vi "Vertical Insert.vi"(4 "Side":T1=enum."right", 8 "error in":errorcluster, 9 "Speed":dbl=10.0, 10 "depth":dbl) -> (0 "error out":errorcluster)   [LabVIEW 2013]
uses:
  ROS/Code/SubVIs/BaxterSide.ctl
  ROS/Code/Console/Servers/ServerSubs/(nist) Arm Globals.vi
  Prim/Fwd Kenimatics - array.vi
  <vilib>/Analysis/Matrix/Numeric/Multiply/Multiply - RM,RM.vi
  Move Matrix.vi
  <vilib>/Analysis/Matrix/NI_Matrix.lvlib
panel:
  in  "MaxAngle":dbl=40.0
  in  "deg/mm":dbl=10.0
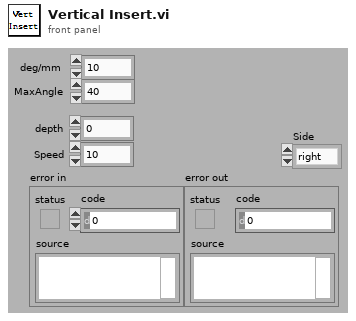
[diagram p1: front panel]
types:
  T1 = typedef "BaxterSide.ctl" = enum16{"left", "right"}
  T2 = cluster{"X":dbl, "Y":dbl, "Z":dbl, "Roll":dbl, "Pitch":dbl, "Yaw":dbl}
  T3 = typedef "NI_Matrix.lvlib/RealMatrix.ctl" = dbl[][]
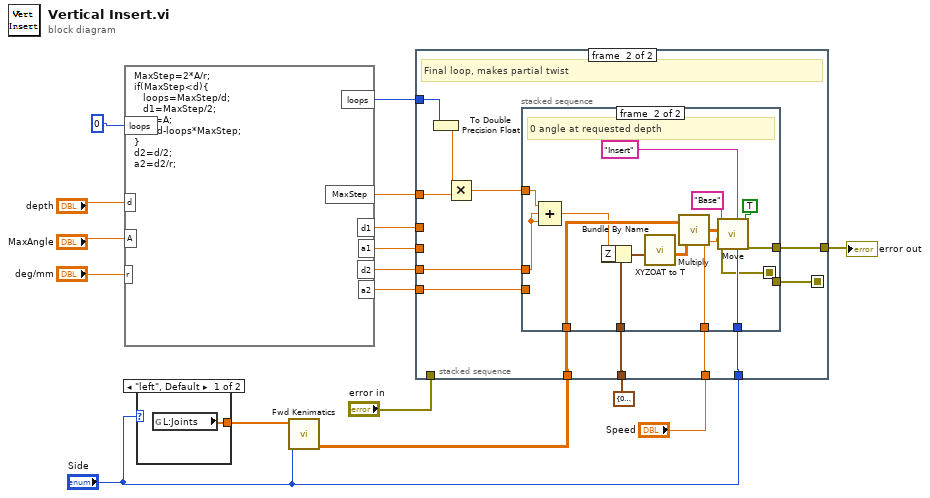
[diagram p0: block diagram]
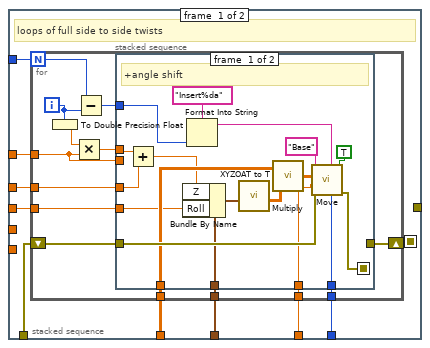
[diagram p2: hidden frame]
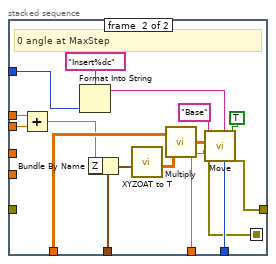
[diagram p3: hidden frame]
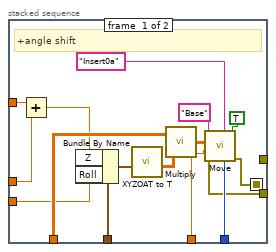
[diagram p4: hidden frame]
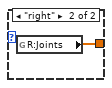
[diagram p5: hidden frame]
diagram:
  n1 = formula code="MaxStep=2*A/r;\nif(MaxStep<d){\n   loops=MaxStep/d;\n   d1=MaxStep/2;\n   a1=A;\n   d=d-loops*MaxStep;\n}\nd2=d/2;\na2=d2/r;"("d"="depth", "A"="MaxAngle", "r"="deg/mm", "loops"=0) -> ("MaxStep"=w5:dbl, "loops"=w13:i32, "d1"=w12:dbl, "a1"=w11:dbl, "d2"=w2:dbl, "a2"=w3:dbl)
  n2 = case shown="\"left\", Default" "Side" {
    tunnel: [w18 w19] -> w17
    frame "left", Default {
      n3 = global read "(nist) Arm Globals.vi" "L:Joints"() -> (w18:dbl[])
    }
    frame "right" {
      n4 = global read "(nist) Arm Globals.vi" "R:Joints"() -> (w19:dbl[])
    }
  }
  n5 = call-poly "Fwd Kenimatics.vi"("Side"="Side", "Joints"=w17) -> ("Matrix"=w9:T3)  [unwired: 8 in, 1 out]
  n6 = stacked-sequence {
    seq-local: [w20 _] -> [_ w83]
    tunnel: w13 -> [w29 w90]
    tunnel: w12 -> [w28 _]
    tunnel: w11 -> [w27 _]
    tunnel: "error in" -> [w26 _]
    tunnel: w9 -> [w25 w84]
    tunnel: T2 {"X"=0.0, "Y"=0.0, "Z"=0.0, "Roll"=0.0, "Pitch"=0.0, "Yaw"=0.0} ("XYZOAT") -> [w24 w81]
    tunnel: "Speed" -> [w23 w82]
    tunnel: "Side" -> [w22 w80]
    tunnel: w5 -> [w21 w89]
    tunnel: w3 -> [_ w87]
    tunnel: w2 -> [_ w86]
    tunnel: [_ w79] -> w1
    frame #0 {
      # "loops of full side to side twists"
      n7 = for {
        N: w29 -> [w32]
        tunnel: w28 -> [w34]
        tunnel: w27 -> [w39]
        shift-right: [w42] -> w20
        shift-left: w26 -> [w43]
        tunnel: w25 -> [w41]
        tunnel: w24 -> [w40]
        tunnel: w23 -> [w38]
        tunnel: w22 -> [w37]
        tunnel: w21 -> [w33]
        i -> [w31]
        n8 = To Double Precision Float(number=w31) -> (double precision float=w36:dbl)
        n9 = Multiply(x=w36, y=w33) -> (x*y=w35:dbl)
        n10 = Subtract(x=w32, y=w31) -> (x-y=w30:i32)
        n11 = stacked-sequence {
          seq-local: [w44 _] -> [_ w66]
          tunnel: w43 -> [w61 _]
          tunnel: w30 -> [w58 w76]
          tunnel: [_ w65] -> w42
          tunnel: w41 -> [w56 w74]
          tunnel: w40 -> [w52 w70]
          tunnel: w39 -> [w48 _]
          tunnel: w38 -> [w50 w68]
          tunnel: w37 -> [w49 w67]
          tunnel: w35 -> [w47 w64]
          tunnel: w34 -> [w46 _]
          tunnel: w33 -> [_ w63]
          frame #0 {
            # "+angle shift"
            n12 = Add(x=w47, y=w46) -> (x+y=w45:dbl)
            n13 = Bundle By Name(cluster=w52, "Z"=w45, "Roll"=w48) -> (w53:T2)
            n14 = Format Into String(format string="Insert%da", w58) -> (resulting string=w57:string)  [unwired: 2 in, 1 out]
            n15 = call "XYZOAT to T.vi"("XYZOAT"=w53) -> ("T"=w54:T3)  [unwired: 10 in]
            n16 = call-poly <vilib>:"Multiply.vi"("Real Matrix B"=w54, "Real Matrix A"=w56) -> ("A * B"=w55:T3)
            n17 = call-poly "Move.vi"("Make Vertical"=TRUE, "Side"=w49, "Label"=w57, "error in"=w61, "Speed (mm/s)"=w50, "Offset"=w55, "Location"="Base") -> ("error out"=w44:errorcluster)  [unwired: 4 in]
          }
          frame #1 {
            # "0 angle at MaxStep"
            n18 = Add(x=w64, y=w63) -> (x+y=w62:dbl)
            n19 = Format Into String(format string="Insert%dc", w76) -> (resulting string=w75:string)  [unwired: 2 in, 1 out]
            n20 = Bundle By Name(cluster=w70, "Z"=w62) -> (w71:T2)
            n21 = call "XYZOAT to T.vi"("XYZOAT"=w71) -> ("T"=w72:T3)  [unwired: 10 in]
            n22 = call-poly <vilib>:"Multiply.vi"("Real Matrix B"=w72, "Real Matrix A"=w74) -> ("A * B"=w73:T3)
            n23 = call-poly "Move.vi"("Make Vertical"=TRUE, "Side"=w67, "Label"=w75, "error in"=w66, "Speed (mm/s)"=w68, "Offset"=w73, "Location"="Base") -> ("error out"=w65:errorcluster)  [unwired: 4 in]
          }
        }
      }
    }
    frame #1 {
      # "Final loop, makes partial twist"
      n24 = To Double Precision Float(number=w90) -> (double precision float=w88:dbl)
      n25 = Multiply(x=w88, y=w89) -> (x*y=w85:dbl)
      n26 = stacked-sequence {
        seq-local: [w93 _] -> [_ w112]
        tunnel: [_ w111] -> w79
        tunnel: w84 -> [w105 w120]
        tunnel: w81 -> [w101 w116]
        tunnel: w87 -> [w97 _]
        tunnel: w82 -> [w99 w114]
        tunnel: w80 -> [w98 w113]
        tunnel: w85 -> [w96 w110]
        tunnel: w86 -> [w95 w108]
        tunnel: w83 -> [w91 _]
        frame #0 {
          # "+angle shift"
          n27 = Add(x=w96, y=w95) -> (x+y=w94:dbl)
          n28 = Bundle By Name(cluster=w101, "Z"=w94, "Roll"=w97) -> (w102:T2)
          n29 = call "XYZOAT to T.vi"("XYZOAT"=w102) -> ("T"=w103:T3)  [unwired: 10 in]
          n30 = call-poly <vilib>:"Multiply.vi"("Real Matrix B"=w103, "Real Matrix A"=w105) -> ("A * B"=w104:T3)
          n31 = call-poly "Move.vi"("Make Vertical"=TRUE, "Side"=w98, "Label"="Insert0a" ("format string"), "error in"=w91, "Speed (mm/s)"=w99, "Offset"=w104, "Location"="Base") -> ("error out"=w93:errorcluster)  [unwired: 4 in]
        }
        frame #1 {
          # "0 angle at requested depth"
          n32 = Compound Arithmetic op=ADD(w110, w108, w108) -> (w109:dbl)
          n33 = Bundle By Name(cluster=w116, "Z"=w109) -> (w117:T2)
          n34 = call "XYZOAT to T.vi"("XYZOAT"=w117) -> ("T"=w118:T3)  [unwired: 10 in]
          n35 = call-poly <vilib>:"Multiply.vi"("Real Matrix B"=w118, "Real Matrix A"=w120) -> ("A * B"=w119:T3)
          n36 = call-poly "Move.vi"("Make Vertical"=TRUE, "Side"=w113, "Label"="Insert" ("format string"), "error in"=w112, "Speed (mm/s)"=w114, "Offset"=w119, "Location"="Base") -> ("error out"=w111:errorcluster)  [unwired: 4 in]
        }
      }
    }
  }
  "error out" <- w1
